vi "LH6HDResponseHandler_inycom.vi"(8 "error in (no error)":errorcluster, 10 "Response":string[](array[string]), 11 "Enum in":enum16{"Tag", "Status"}(ring)) -> (0 "error out":errorcluster, 2 "Enum out":T1(ring), 3 "String":string)   [LabVIEW 2015]
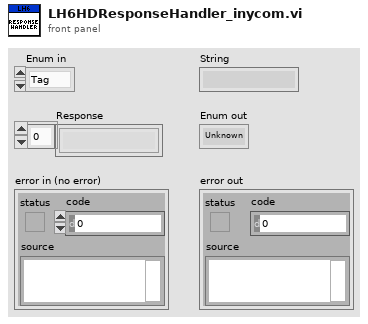
[diagram p1: front panel]
types:
  T1 = enum16{"Unknown", "Estado OK", "Ocupado", "Inhibit OK", "Waiting", "Reset"}
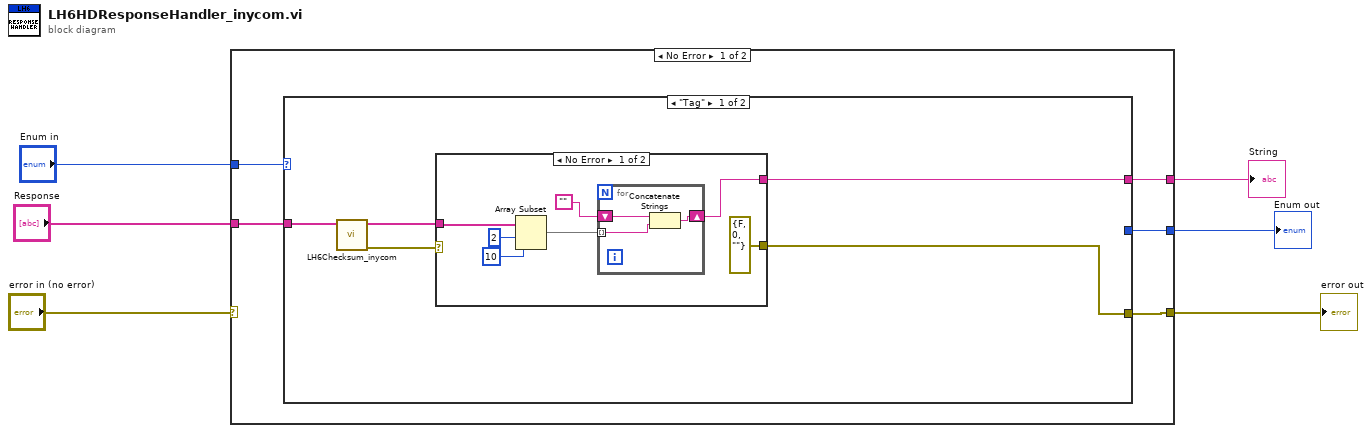
[diagram p0: block diagram]
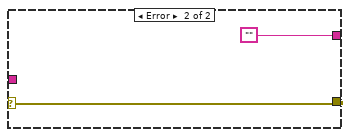
[diagram p2: hidden frame]
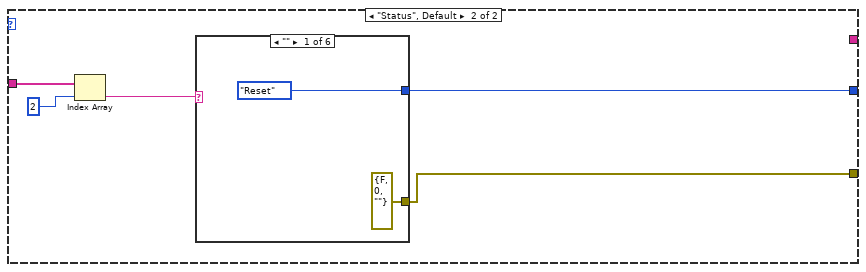
[diagram p3: hidden frame]
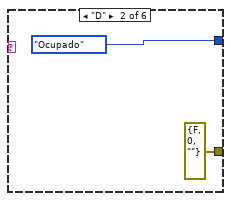
[diagram p4: hidden frame]
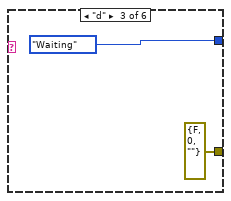
[diagram p5: hidden frame]
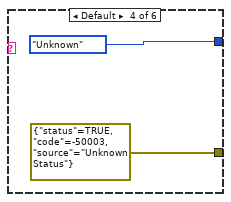
[diagram p6: hidden frame]
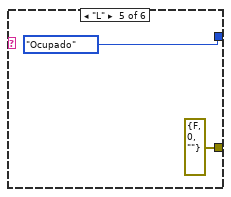
[diagram p7: hidden frame]
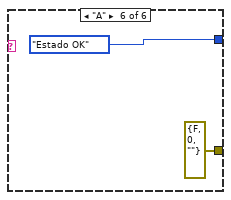
[diagram p8: hidden frame]
diagram:
  n1 = case shown="No Error" "error in (no error)" {
    selector: "error in (no error)" -> [_ w46]
    tunnel: [w8 w46] -> w2
    tunnel: "Enum in" -> [w11 _]
    tunnel: "Response" -> [w10 _]
    tunnel: [w9 _] -> w5
    tunnel: [w7 _] -> w6
    frame No Error {
      n2 = case shown="\"Tag\"" w11 {
        tunnel: w10 -> [w16 w32]
        tunnel: [w13 _] -> w9
        tunnel: [w12 w30] -> w8
        tunnel: [_ w29] -> w7
        frame "Tag" {
          n3 = call "LH6Checksum_inycom.vi"("Data in"=w16) -> ("error out"=w15:errorcluster, "Data out"=w14:string[])  [unwired: 9 in]
          n4 = case shown="No Error" w15 {
            selector: w15 -> [_ w27]
            tunnel: w14 -> [w21 _]
            tunnel: [w18 ""] -> w13
            tunnel: [errorcluster {"status"=FALSE, "code"=0, "source"=""} ("error IO") w27] -> w12
            frame No Error {
              n5 = Array Subset(array=w21, index=2, length=10) -> (w20:string[])
              n6 = for {
                tunnel: w20 -> [w26] mode=indexing
                shift-right: [w25] -> w18
                shift-left: "" -> [w24]
                n7 = Concatenate Strings(w24, w26) -> (w25:string)
              }
            }
            frame Error {
            }
          }
        }
        frame "Status", Default {
          n8 = Index Array(array=w32, index=2) -> (element=w31:string)
          n9 = case shown="\"\"" w31 {
            tunnel: [T1."Reset" T1."Ocupado" T1."Waiting" T1."Unknown" T1."Ocupado" T1."Estado OK"] -> w29
            tunnel: [errorcluster {"status"=FALSE, "code"=0, "source"=""} ("error IO") errorcluster {"status"=FALSE, "code"=0, "source"=""} ("error IO") errorcluster {"status"=FALSE, "code"=0, "source"=""} ("error IO") errorcluster {"status"=TRUE, "code"=-50003, "source"="Unknown Status"} ("error IO") errorcluster {"status"=FALSE, "code"=0, "source"=""} ("error IO") errorcluster {"status"=FALSE, "code"=0, "source"=""} ("error IO")] -> w30
            frame "" {
            }
            frame "D" {
            }
            frame "d" {
            }
            frame Default {
            }
            frame "L" {
            }
            frame "A" {
            }
          }
        }
      }
    }
    frame Error {
    }
  }
  "Enum out" <- w6
  "String" <- w5
  "error out" <- w2
